vi "Check Response.vi"(8 "Error In":errorcluster, 10 "Read Buffer":string, 11 "VISA resource":refnum<visa-resource-name>) -> (0 "error out":errorcluster, 2 "Filtered Response":string, 3 "VISA resource  out":refnum<visa-resource-name>)   [LabVIEW 2010, in "FEM-03.lvlib"]
uses:
  FEM-03.lvlib
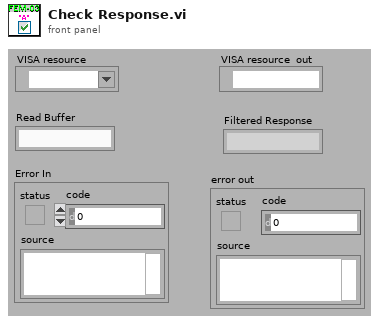
[diagram p1: front panel]
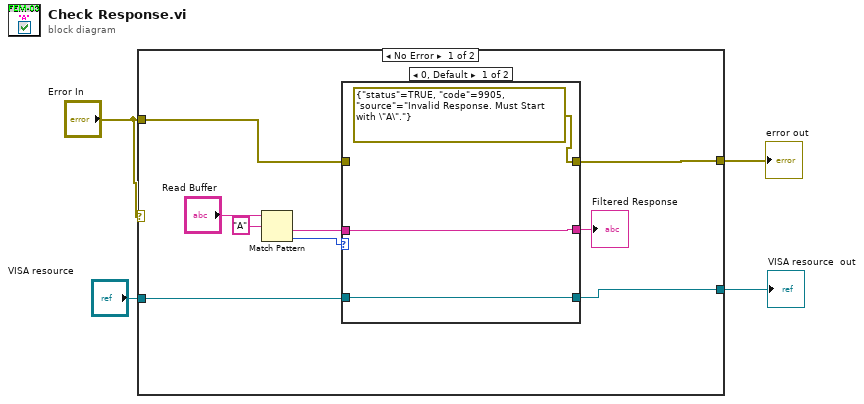
[diagram p0: block diagram]
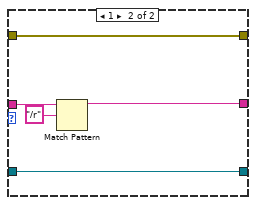
[diagram p2: hidden frame]
diagram:
  n1 = case shown="No Error" "Error In" {
    tunnel: [w12 w23] -> w4
    tunnel: "Error In" -> [w11 w23]
    tunnel: "VISA resource" -> [w6 w22]
    tunnel: [w5 w22] -> w1
    frame No Error {
      n2 = Match Pattern(string="Read Buffer", regular expression="A") -> (after substring=w13:string, offset past match=w10:i32)  [unwired: 1 in, 2 out]
      n3 = case shown="0, Default" w10 {
        tunnel: w6 -> [w16 w21]
        tunnel: [w16 w21] -> w5
        tunnel: w11 -> [_ w20]
        tunnel: [errorcluster {"status"=TRUE, "code"=9905, "source"="Invalid Response. Must Start with \"A\"."} ("error out") w20] -> w12
        tunnel: w13 -> [w15 w18]
        tunnel: [w15 w17] -> w7
        frame 0, Default {
        }
        frame 1 {
          n4 = Match Pattern(string=w18, regular expression="/r") -> (before substring=w17:string)  [unwired: 1 in, 3 out]
        }
      }
      "Filtered Response" <- w7
    }
    frame Error {
    }
  }
  "error out" <- w4
  "VISA resource  out" <- w1
